vi "Lev-Mar abx_mod_v05.vi"(0 "X":dbl[](array[numeric]) format="%.2f", 1 "formula":string, 2 "Y":dbl[](array[numeric]) format="%.2f", 3 "Coefficients":dbl[](array[numeric]) format="%.2f", 5 "W":dbl[](array[numeric]) format="%.2f") -> (6 "Alpha":dbl[][](array[numeric]) format="%.2f", 7 "Beta":dbl[](array[numeric]) format="%.2f", 8 "chiSqr":dbl format="%.2f")   [LabVIEW 2010]
panel:
  # "Array Lev-Mar\nabx"
  # "Array modifications by\nChristian Altenbach\ncaltenba@ucla.edu"
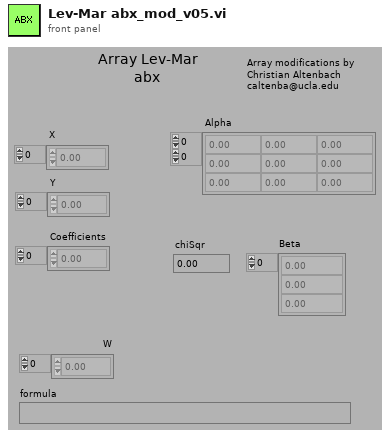
[diagram p1: front panel]
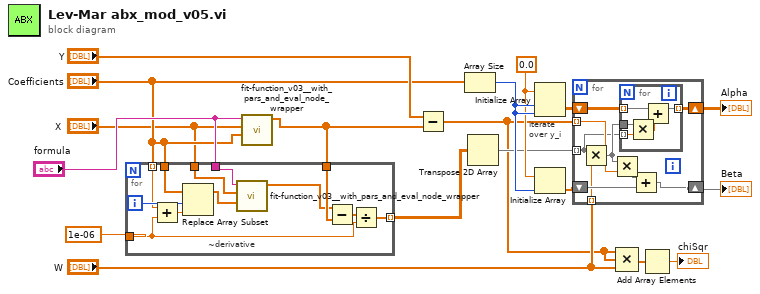
[diagram p0: block diagram]
diagram:
  w15 = 0.0
  # "iterate\nover y_i"
  n1 = call "fit-function_v03__with_pars_and_eval_node_wrapper.vi"("coefficients"="Coefficients", "x"="X", "formula"="formula") -> ("y"=w1:dbl[])  [unwired: 7 in, 1 out]
  n2 = for {
    tunnel: [w26] -> w6 mode=indexing
    tunnel: "Coefficients" -> [w27] mode=indexing
    tunnel: "Coefficients" -> [w25]
    tunnel: 1e-06 -> [w24]
    tunnel: w1 -> [w23]
    tunnel: "formula" -> [w20]
    tunnel: "X" -> [w21]
    i -> [w28]
    # "~derivative"
    n3 = Add(x=w27, y=w24) -> (x+y=w29:dbl)
    n4 = Replace Array Subset(array=w25, new element=w29, index=w28) -> (w22:dbl[])
    n5 = call "fit-function_v03__with_pars_and_eval_node_wrapper.vi"("coefficients"=w22, "x"=w21, "formula"=w20) -> ("y"=w19:dbl[])  [unwired: 7 in, 1 out]
    n6 = Subtract(x=w19, y=w23) -> (x-y=w30:dbl[])
    n7 = Divide(x=w30, y=w24) -> (x/y=w26:dbl[])
  }
  n8 = Subtract(x="Y", y=w1) -> (x-y=w5:dbl[])
  n9 = Array Size(array="Coefficients") -> (size(s)=w18:i32)
  n10 = Transpose 2D Array(2D array=w6) -> (transposed array=w8:dbl[][])
  n11 = Initialize Array(w15, w18, w18) -> (w16:dbl[][])
  n12 = Initialize Array(w15, w18) -> (w17:dbl[])
  n13 = for {
    shift-right: [w37] -> w14
    shift-left: w17 -> [w39]
    shift-right: [w35] -> w13
    shift-left: w16 -> [w36]
    tunnel: w8 -> [w31] mode=indexing
    tunnel: w5 -> [w34] mode=indexing
    tunnel: "W" -> [w33] mode=indexing
    n14 = Multiply(x=w31, y=w33) -> (x*y=w32:dbl[])
    n15 = Multiply(x=w32, y=w34) -> (x*y=w38:dbl[])
    n16 = for {
      tunnel: w32 -> [w44]
      tunnel: w36 -> [w43] mode=indexing
      tunnel: [w41] -> w35 mode=indexing
      tunnel: w31 -> [w40] mode=indexing
      n17 = Multiply(x=w44, y=w40) -> (x*y=w42:dbl[])
      n18 = Add(x=w43, y=w42) -> (x+y=w41:dbl[])
    }
    n19 = Add(x=w38, y=w39) -> (x+y=w37:dbl[])
  }
  "Alpha" <- w13
  "Beta" <- w14
  n20 = Compound Arithmetic op=MULTIPLY(w5, w5, "W") -> (w11:dbl[])
  n21 = Add Array Elements(numeric array=w11) -> (sum=→"chiSqr":dbl)
